vi "Compare Variants.vi"(6 "Delta":variant, 8 "error in (no error)":errorcluster, 9 "Actual":variant, 10 "Expected":variant) -> (0 "error out":errorcluster, 2 "Equal?":bool)   [LabVIEW 2020, in "LUnit Test Case.lvclass"]
uses:
  LUnit Test Case.lvclass
  a05a4bce-3527-4973-9d51-9cb2f6f1166e.vi
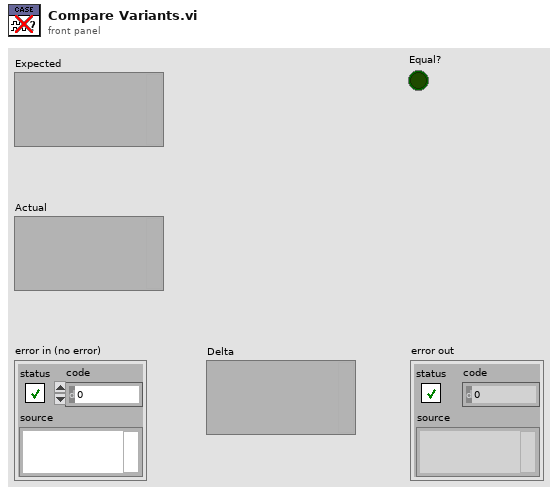
[diagram p1: front panel]
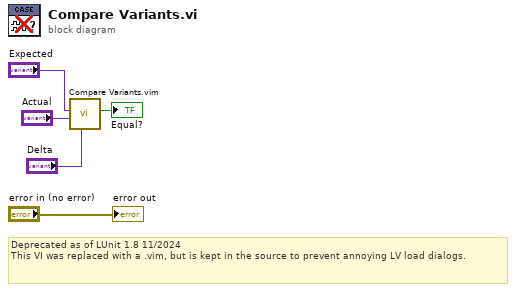
[diagram p0: block diagram]
diagram:
  # "Deprecated as of LUnit 1.8 11/2024\nThis VI was replaced with a .vim, but is kept in the source to prevent annoying LV load dialogs."
  n1 = call "Compare Variants.vim"("Delta"="Delta", "Actual"="Actual", "Expected"="Expected") -> ("Equal?"=→"Equal?":bool)  [unwired: 8 in]
  "error out" <- "error in (no error)"
